vi "Read.vi"(8 "error in (no error)":errorcluster, 11 "Enum in":refnum<class "Enum.lvclass">) -> (0 "error out":errorcluster, 1 "Enum Alias":string, 2 "Enum Index":u32, 3 "Enum out":refnum<class "Enum.lvclass">)   [LabVIEW 2020, in "Data.lvlib" / "Enum.lvclass"]
doc: "Read Enum."
uses:
  Enum.lvclass
  Enum.lvclass/Enum.ctl
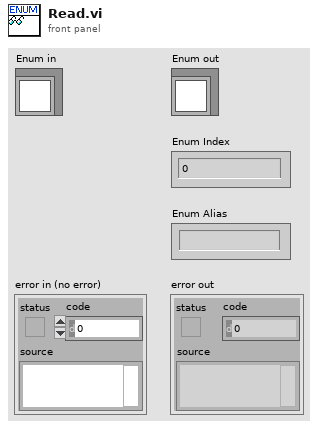
[diagram p1: front panel]
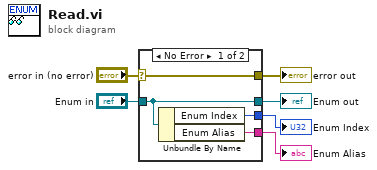
[diagram p0: block diagram]
diagram:
  n1 = case shown="No Error" "error in (no error)" {
    selector: "error in (no error)" -> [w10 w11]
    tunnel: [w10 w11] -> w5
    tunnel: [w9 w12] -> w3
    tunnel: "Enum in" -> [w9 w12]
    tunnel: [w8 _] -> w2
    tunnel: [w7 _] -> w1
    frame No Error {
      n2 = Unbundle By Name(w9) -> ("Enum Index"=w8:u32, "Enum Alias"=w7:string)
    }
    frame Error {
    }
  }
  "error out" <- w5
  "Enum out" <- w3
  "Enum Alias" <- w1
  "Enum Index" <- w2
